vi "verifyThreshold.vi"(0 "#Peaks":i32, 1 "valesAmplitude":dbl[](array[numeric]), 2 "peaksAmplitude":dbl[](array[numeric]), 3 "Error In":errorcluster, 4 "threshold":dbl) -> (5 "passThreshold":i32[](array[numeric]), 6 "Error Out":errorcluster)   [LabVIEW 2015]
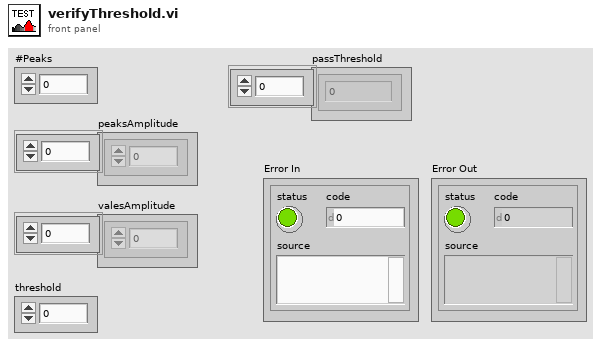
[diagram p1: front panel]
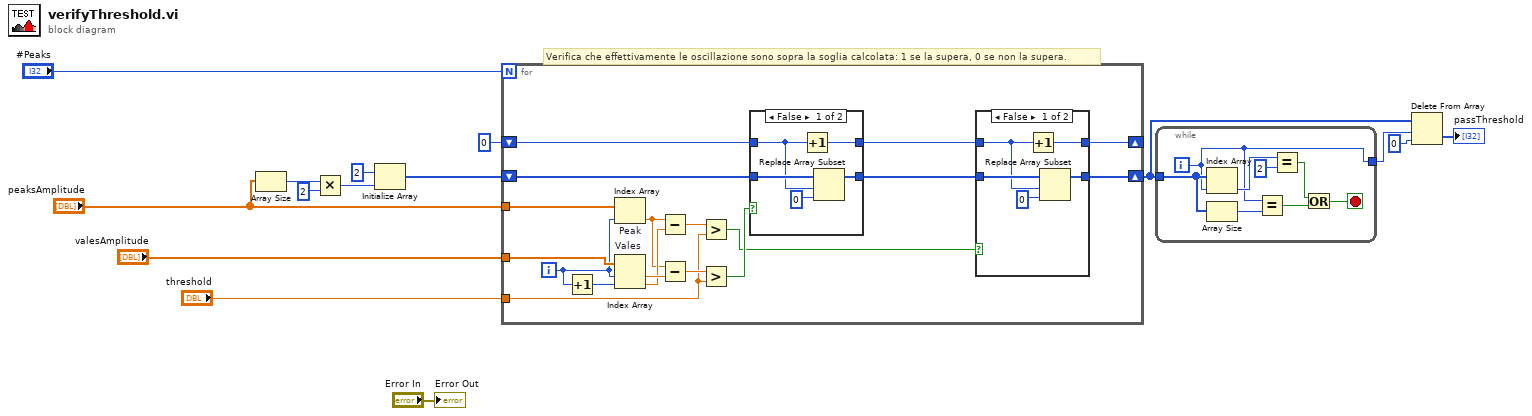
[diagram p0: block diagram]
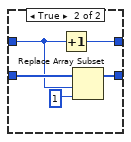
[diagram p2: hidden frame]
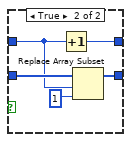
[diagram p3: hidden frame]
diagram:
  # "Verifica che effettivamente le oscillazione sono sopra la soglia calcolata: 1 se la supera, 0 se non la supera."
  n1 = Array Size(array="peaksAmplitude") -> (size(s)=w6:i32)
  n2 = Multiply(x=w6, y=2) -> (x*y=w9:i32)
  n3 = Initialize Array(2 ("element"), w9) -> (w10:i32[])
  n4 = for {
    N: "#Peaks" -> [_]
    tunnel: "peaksAmplitude" -> [w33]
    tunnel: "valesAmplitude" -> [w26]
    tunnel: "threshold" -> [w30]
    shift-right: [w16] -> w12
    shift-left: w10 -> [w23]
    shift-right: [w18] -> _
    shift-left: 0 -> [w20]
    i -> [w22]
    n5 = Increment(x=w22) -> (x+1=w25:i32)
    n6 = Index Array "Peak"(array=w33, index=w22) -> (element=w27:dbl)
    n7 = Index Array "Vales"(array=w26, index #1=w22, index #2=w25) -> (element #1=w29:dbl, element #2=w28:dbl)
    n8 = Subtract(x=w27, y=w28) -> (x-y=w32:dbl)
    n9 = Subtract(x=w27, y=w29) -> (x-y=w31:dbl)
    n10 = Greater?(x=w32, y=w30) -> (0:w17:bool)
    n11 = Greater?(x=w31, y=w30) -> (0:w24:bool)
    n12 = case shown="False" w24 {
      tunnel: w23 -> [w48 w53]
      tunnel: [w46 w51] -> w21
      tunnel: w20 -> [w45 w49]
      tunnel: [w44 w50] -> w19
      frame False {
        n13 = Increment(x=w45) -> (x+1=w44:i32)
        n14 = Replace Array Subset(array=w48, new element=0 ("new element/subarray"), index=w45) -> (w46:i32[])
      }
      frame True {
        n15 = Increment(x=w49) -> (x+1=w50:i32)
        n16 = Replace Array Subset(array=w53, new element=1 ("new element/subarray"), index=w49) -> (w51:i32[])
      }
    }
    n17 = case shown="False" w17 {
      tunnel: w21 -> [w38 w42]
      tunnel: w19 -> [w35 w41]
      tunnel: [w37 w43] -> w18
      tunnel: [w36 w39] -> w16
      frame False {
        n18 = Increment(x=w35) -> (x+1=w37:i32)
        n19 = Replace Array Subset(array=w38, new element=0 ("new element/subarray"), index=w35) -> (w36:i32[])
      }
      frame True {
        n20 = Increment(x=w41) -> (x+1=w43:i32)
        n21 = Replace Array Subset(array=w42, new element=1 ("new element/subarray"), index=w41) -> (w39:i32[])
      }
    }
  }
  n22 = while {
    tunnel: w12 -> [w58]
    tunnel: [w54] -> w14
    i -> [w54]
    stop <- w55 stop-if-true
    n23 = Index Array(array=w58, index=w54) -> (element=w61:i32)
    n24 = Array Size(array=w58) -> (size(s)=w57:i32)
    n25 = Equal?(x=w54, y=w57) -> (x = y?=w56:bool)
    n26 = Equal?(x=w61, y=2) -> (x = y?=w59:bool)
    n27 = Or(x=w59, y=w56) -> (x .or. y?=w55:bool)
  }
  n28 = Delete From Array(array=w12, length=w14, index=0) -> (deleted portion=→"passThreshold":i32[])  [unwired: 1 out]
  "Error Out" <- "Error In"
